vi "L0_SumnAdds_File_Appender.vi"(0 "Vin":dbl, 1 "CH":dbl, 2 "Att":dbl, 3 "IbClip":dbl=63.0, 4 "Clip":dbl=1.0, 5 "Vmeas":dbl, 7 "file path (dialog if empty)":path) -> ()   [LabVIEW 2009]
uses:
  <vilib>/Utility/file.llb/Write To Spreadsheet File (string).vi
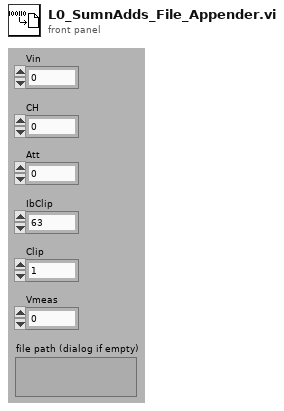
[diagram p1: front panel]
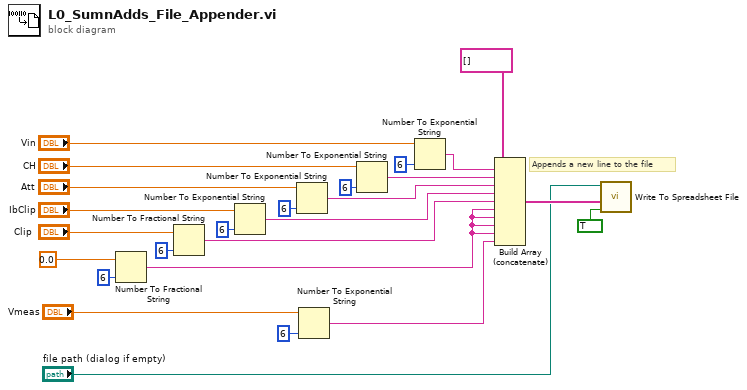
[diagram p0: block diagram]
diagram:
  # "Appends a new line to the file"
  n1 = Number To Fractional String(number=0.0, precision (6)=i16 6) -> (F-format string=w1:string)  [unwired: 2 in]
  n2 = Number To Fractional String(number="Clip", precision (6)=i16 6) -> (F-format string=w18:string)  [unwired: 2 in]
  n3 = Number To Exponential String(number="IbClip", precision (6)=i16 6) -> (E-format string=w22:string)  [unwired: 2 in]
  n4 = Number To Exponential String(number="Att", precision (6)=i16 6) -> (E-format string=w24:string)  [unwired: 2 in]
  n5 = Number To Exponential String(number="Vmeas", precision (6)=i16 6) -> (E-format string=w10:string)  [unwired: 2 in]
  n6 = Number To Exponential String(number="CH", precision (6)=i16 6) -> (E-format string=w25:string)  [unwired: 2 in]
  n7 = Number To Exponential String(number="Vin", precision (6)=i16 6) -> (E-format string=w17:string)  [unwired: 2 in]
  n8 = Build Array (concatenate)(string[] [] ("array"), w17, w25, w24, w22, w18, w1, w1, w1, w1, w10) -> (w13:string[])
  n9 = call-poly <vilib>:"Write To Spreadsheet File.vi"("append to file? (new file:F)"=TRUE, "1D data"=w13, "file path (dialog if empty)"="file path (dialog if empty)") -> ()  [unwired: 5 in, 1 out]
